vi "state graph.vi"(4 "Clear graph":bool, 5 "sensor to plot":i32[](listbox), 6 "history length":u16=1000 min=1, 7 "graph update interval":sgl=1.0 min=0.001 format="%.2f") -> (0 "Sensor Data Smoothed":T1 {"Sensor array"."scaled" format="%.2f"; "Sensor array"."voltage" format="%.4f"; "Time" format="%<%I:%M:%S%2u %p\n%m/%d/%Y>T"}, 1 "state graph":cluster{dbl[], dbl[]}, 3 "sensor graph array":cluster{dbl[], dbl[]}[](array[cluster]))   [LabVIEW 2015]
uses:
  TCP DAQ/Sensor data.ctl
  DAQ configuration/sensor cluster.ctl
  DAQ configuration/Sensor buffer command.ctl
  logic buffer cmd.ctl
  calibration/Shared Data/share data command.ctl
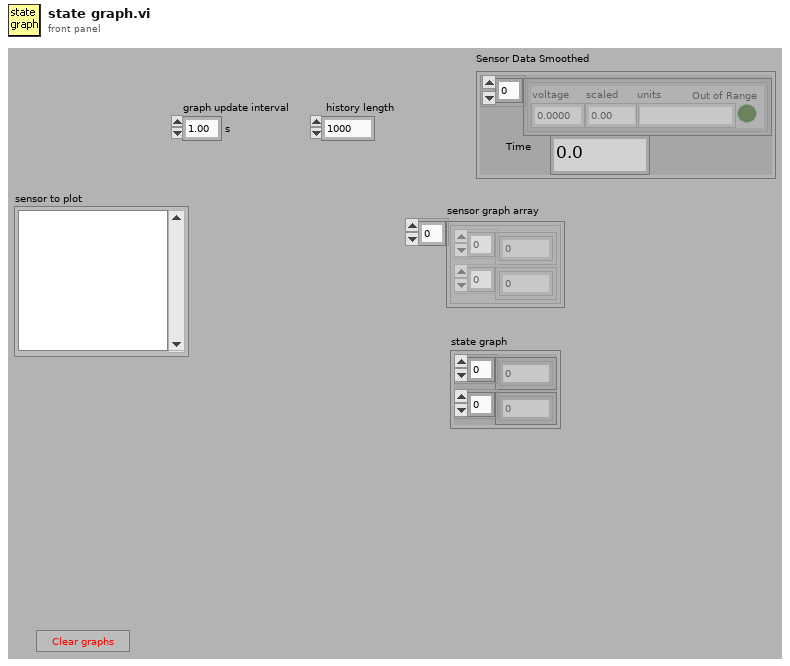
[diagram p1: front panel]
types:
  T1 = typedef "Sensor data.ctl" = cluster{" Sensor array":T2[], "Time":dbl}
  T2 = typedef "sensor cluster.ctl" = cluster{"voltage":sgl, "scaled":sgl, "units":string, "Out of Range":bool}
  T3 = typedef "share data command.ctl" = enum16{"Initialize from ini", "Update ini", "Write data", "Read data", "List my data", "List shared data", "Close"}
  T4 = typedef "logic buffer cmd.ctl" = enum16{"read", "write ouput settings", "write rules", "write setpoints", "write output descriptions", "write all", "calculate setpoints", "save", "open", "Load all setpoint code", "Load one setpoint code", "Configure one setpoint code"}
  T5 = typedef "Sensor buffer command.ctl" = enum16{"read average", "read recent", "read all", "write", "set buffer size", "Read channel config", "Write channel config", "clear"}
  T6 = typedef "variable setpoint.ctl" = cluster{"name":string, "unit":string, "value":dbl, "Type":enum16{"Constant", "Variable"}, "variable":cluster{"selected sensors":i32[], "selected set points":i32[], "VI":path, "Data average interval":T7, "code ref":T8}}
  T7 = typedef "data ave interval.ctl" = dbl
  T8 = typedef "type specifier for control code.ctl" = refnum<vi>
  T9 = typedef "Plant state.ctl" = u16
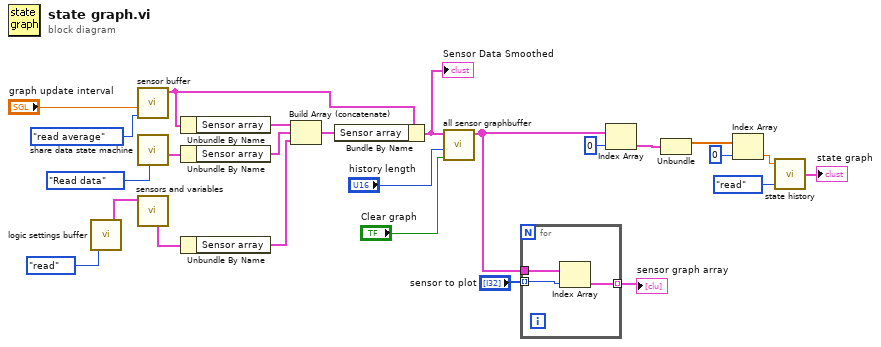
[diagram p0: block diagram]
diagram:
  n1 = call "logic settings buffer.vi"("command"=logic_buffer_cmd."read") -> ("Set Points out"=w16:T6[])  [unwired: 11 in, 7 out]
  n2 = call "sensor buffer.vi"("command"=Sensor_buffer_command."read average", "smooth interval (s)"="graph update interval") -> ("Calibrated data"=w15:T1)  [unwired: 5 in, 4 out]
  n3 = call "share data state machine.vi"("Share data command"=share_data_command."Read data") -> ("Data from shared sources"=w9:T1)  [unwired: 4 in, 6 out]
  n4 = call "sensors and variables.vi"("S P & V definitions"=w16) -> ("Calibrated data"=w6:T1)  [unwired: 6 in, 4 out]
  n5 = Unbundle By Name(w15) -> ("Sensor array"=w8:T2[])
  n6 = Unbundle By Name(w9) -> ("Sensor array"=w7:T2[])
  n7 = Unbundle By Name(w6) -> ("Sensor array"=w5:T2[])
  n8 = Build Array (concatenate)(w8, w7, w5) -> (w14:T2[])
  n9 = Bundle By Name(cluster=w15, "Sensor array"=w14) -> (w13:T1)
  "Sensor Data Smoothed" <- w13
  n10 = call "all sensor graphbuffer.vi"("Reset"="Clear graph", "history length"="history length", "Sensor Data"=w13) -> ("Multiplot graph data"=w3:cluster{dbl[], dbl[]}[])  [unwired: 6 in, 2 out]
  n11 = for {
    tunnel: "sensor to plot" -> [w28] mode=indexing
    tunnel: w3 -> [w27]
    tunnel: [w26] -> w1 mode=indexing
    n12 = Index Array(array=w27, index=w28) -> (element=w26:cluster{dbl[], dbl[]})
  }
  "sensor graph array" <- w1
  n13 = Index Array(array=w3, index=0) -> (element=w20:cluster{dbl[], dbl[]})
  n14 = Unbundle(w20) -> (w23:dbl[])  [unwired: 1 out]
  n15 = Index Array(array=w23, index=0) -> (element=w21:dbl)
  n16 = call "state history.vi"("command"=enum16{"write", "read", "reset"}."read", "Time"=w21) -> ("state history"=→"state graph":cluster{dbl[], T9[]})  [unwired: 1 in]
